vi "addNewParagraph.vi"(8 "error in (no error)":errorcluster, 10 "New Paragraph":refnum<class "xwpfParagraph.lvclass">, 11 "xwpfDocument in":refnum<class "xwpfDocument.lvclass">) -> (0 "error out":errorcluster, 3 "xwpfDocument out":refnum<class "xwpfDocument.lvclass">)   [LabVIEW 2017, in "Word_Specific.lvlib" / "xwpfDocument.lvclass"]
uses:
  xwpfDocument.lvclass
  xwpfParagraph/xwpfParagraph.lvclass
  xwpfDocument.lvclass/xwpfDocument.ctl
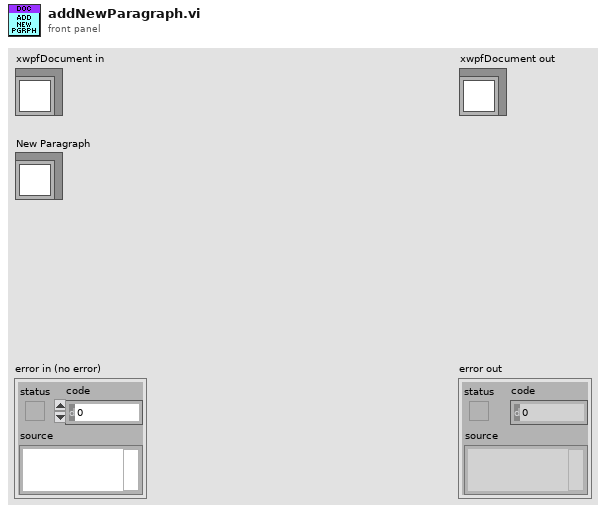
[diagram p1: front panel]
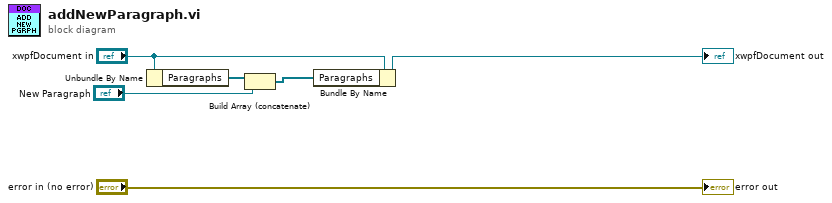
[diagram p0: block diagram]
diagram:
  n1 = Unbundle By Name("xwpfDocument in") -> ("Paragraphs"=w4:refnum<class "xwpfParagraph.lvclass">[])
  n2 = Build Array (concatenate)(w4, "New Paragraph") -> (w3:refnum<class "xwpfParagraph.lvclass">[])
  n3 = Bundle By Name(cluster="xwpfDocument in", "Paragraphs"=w3) -> (→"xwpfDocument out":refnum<class "xwpfDocument.lvclass">)
  "error out" <- "error in (no error)"
